vi "InitDataQ.vi"(8 "ErrorIn(No Error)":errorcluster caption="entrée d'erreur (pas d'erreur)", 11 "Interface.lvclass":refnum<class "Interface.lvclass">) -> (0 "sortie d'erreur":errorcluster, 3 "Interface.lvclass Out":refnum<class "Interface.lvclass">)   [LabVIEW 2019, in "Interface.lvclass"]
uses:
  Interface.lvclass
  Interface.lvclass/Interface.ctl
  <userlib>/GenProg/ArrayTo1DString.vi
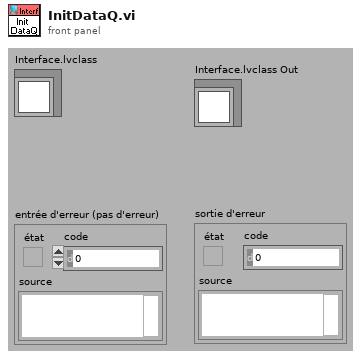
[diagram p1: front panel]
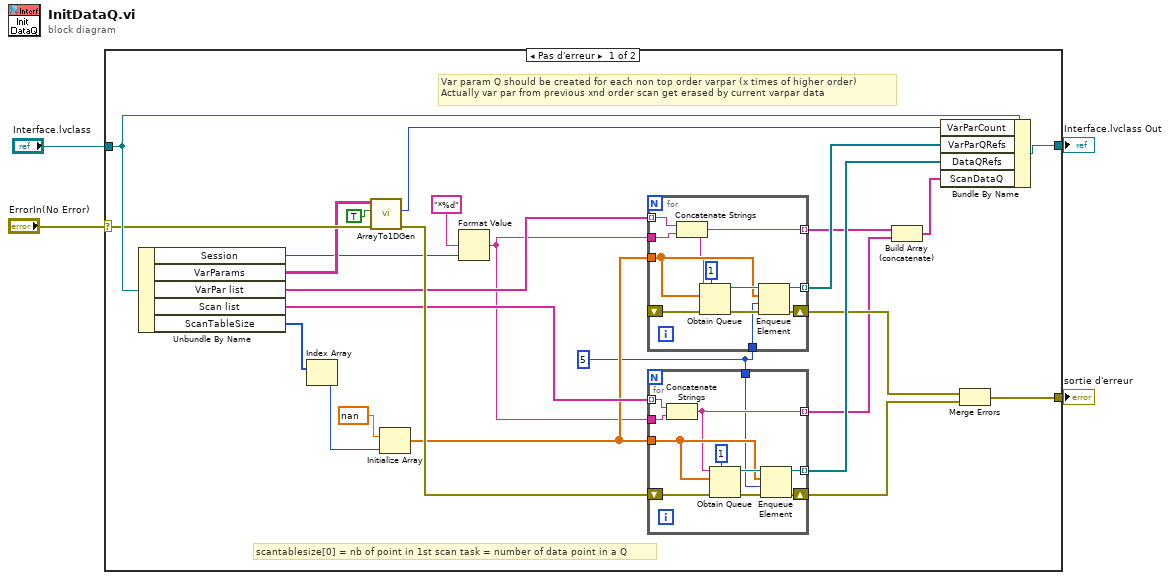
[diagram p0: block diagram]
diagram:
  n1 = case shown="Pas d'erreur" "ErrorIn(No Error)" {
    selector: "ErrorIn(No Error)" -> [w22 w53]
    tunnel: [w5 w53] -> w3
    tunnel: "Interface.lvclass" -> [w27 w52]
    tunnel: [w25 w52] -> w2
    frame No Error {
      w6 = 5 ("timeout en ms (-1)")
      # "Var param Q should be created for each non top order varpar (x times of higher order) \nActually var par from previous xnd order scan get erased by current varpar data"
      # "scantablesize[0] = nb of point in 1st scan task = number of data point in a Q"
      n2 = Unbundle By Name(w27) -> ("Session"=w12:i32, "VarParams"=w20:string[][], "VarPar list"=w13:string[], "Scan list"=w17:string[], "ScanTableSize"=w24:i32[])
      n3 = Index Array(array=w24) -> (element=w18:i32)  [unwired: 1 in]
      n4 = call-poly <userlib>:"ArrayTo1DGen.vi"("ErrorIn(No Error)"=w22, "DelArrEnd(F)"=TRUE ("DelArrEnd"), "tableau"=w20) -> ("sortie d'erreur"=w21:errorcluster, "Size"=w19:i32)  [unwired: 6 in, 1 out]
      n5 = Initialize Array(nan ("élément"), w18) -> (w16:dbl[])
      n6 = Format Value(format string="*%d" ("chaîne (\"\")"), value (0)=w12) -> (output string=w10:string)  [unwired: 1 in]
      n7 = for {
        tunnel: [w37] -> w14 mode=indexing
        tunnel: w16 -> [w36]
        shift-right: [w38] -> w15
        shift-left: _ -> [w35]
        tunnel: w13 -> [w32] mode=indexing
        tunnel: w10 -> [w33]
        tunnel: [w31] -> w9 mode=indexing
        tunnel: w6 -> [w30]
        n8 = Concatenate Strings(w32, w33) -> (w31:string)
        n9 = Obtain Queue(max queue size (-1, unlimited)=1 ("taille max de la file d'attente (-1, non limitée)"), name (unnamed)=w31, element data type=w36, error in (no error)=w35) -> (queue out=w39:refnum<queue>, error out=w40:errorcluster)  [unwired: 1 in, 1 out]
        n10 = Enqueue Element(queue=w39, element=w36, timeout in ms (-1)=w30, error in (no error)=w40) -> (queue out=w37:refnum<queue>, error out=w38:errorcluster)  [unwired: 1 out]
      }
      n11 = for {
        tunnel: [w48] -> w26 mode=indexing
        tunnel: w16 -> [w47]
        shift-right: [w49] -> w29
        shift-left: w21 -> [w46]
        tunnel: w17 -> [w44] mode=indexing
        tunnel: w10 -> [w43]
        tunnel: [w42] -> w8 mode=indexing
        tunnel: w6 -> [w41]
        n12 = Concatenate Strings(w44, w43) -> (w42:string)
        n13 = Obtain Queue(max queue size (-1, unlimited)=1 ("taille max de la file d'attente (-1, non limitée)"), name (unnamed)=w42, element data type=w47, error in (no error)=w46) -> (queue out=w50:refnum<queue>, error out=w51:errorcluster)  [unwired: 1 in, 1 out]
        n14 = Enqueue Element(queue=w50, element=w47, timeout in ms (-1)=w41, error in (no error)=w51) -> (queue out=w48:refnum<queue>, error out=w49:errorcluster)  [unwired: 1 out]
      }
      n15 = Build Array (concatenate)(w9, w8) -> (w7:string[])
      n16 = Bundle By Name(cluster=w27, "VarParCount"=w19, "VarParQRefs"=w14, "DataQRefs"=w26, "ScanDataQ"=w7) -> (w25:refnum<class "Interface.lvclass">)
      n17 = Merge Errors(w15, w29) -> (w5:errorcluster)
    }
    frame Error {
    }
  }
  "sortie d'erreur" <- w3
  "Interface.lvclass Out" <- w2
